vi "registerCommands.vi"(8 "error in (no error)":errorcluster, 11 "SAL_Listener in":refnum<class "SAL_Listener.lvclass">) -> (0 "error out":errorcluster, 3 "SAL_Listener out":refnum<class "SAL_Listener.lvclass">)   [LabVIEW 2016, in "SAL_Listener.lvclass"]
uses:
  SAL_Listener.lvclass
  SAL_Listener.lvclass/SAL_Listener.ctl
  SALLV_dome/SALLV_dome.lvlib
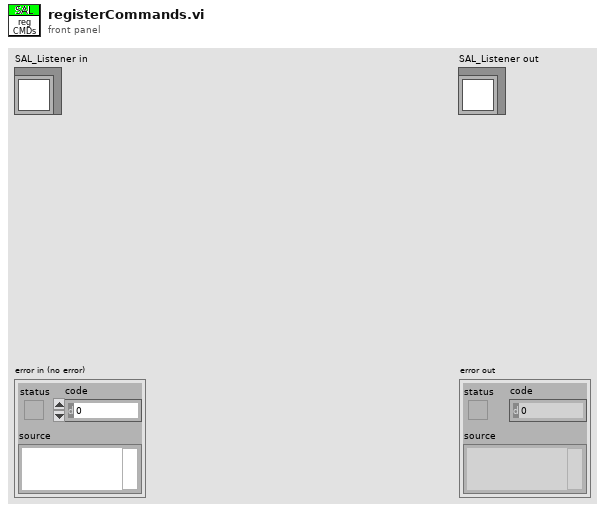
[diagram p1: front panel]
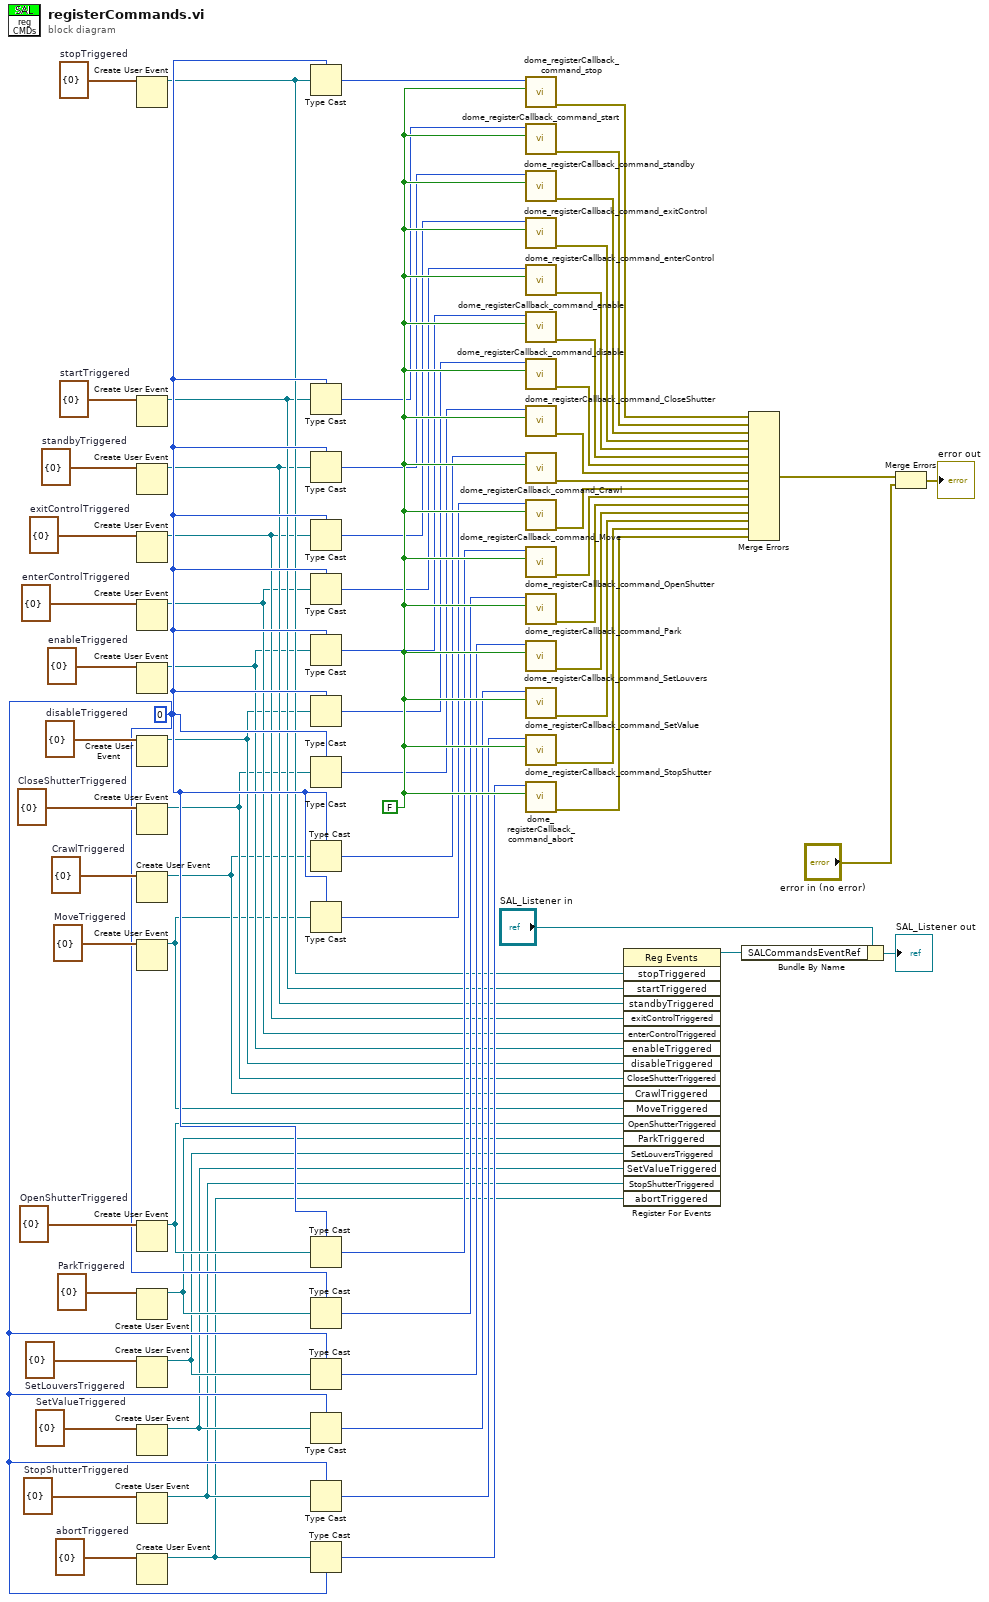
[diagram p0: block diagram]
diagram:
  w55 = 0 ("handle")
  w56 = FALSE
  w57 = cluster{"data":i32} {"data"=0}  # abortTriggered
  w59 = cluster{"data":i32} {"data"=0}  # SetValueTriggered
  w58 = cluster{"data":i32} {"data"=0}  # StopShutterTriggered
  w60 = cluster{"data":i32} {"data"=0}  # SetLouversTriggered
  w61 = cluster{"data":i32} {"data"=0}  # ParkTriggered
  w62 = cluster{"data":i32} {"data"=0}  # OpenShutterTriggered
  w63 = cluster{"data":i32} {"data"=0}  # MoveTriggered
  w64 = cluster{"data":i32} {"data"=0}  # CrawlTriggered
  w65 = cluster{"data":i32} {"data"=0}  # CloseShutterTriggered
  w66 = cluster{"data":i32} {"data"=0}  # disableTriggered
  w67 = cluster{"data":i32} {"data"=0}  # enableTriggered
  w68 = cluster{"data":i32} {"data"=0}  # enterControlTriggered
  w69 = cluster{"data":i32} {"data"=0}  # exitControlTriggered
  w70 = cluster{"data":i32} {"data"=0}  # standbyTriggered
  w71 = cluster{"data":i32} {"data"=0}  # startTriggered
  w72 = cluster{"data":i32} {"data"=0}  # stopTriggered
  n1 = Create User Event(user event datatype=w72) -> (user event=w19:refnum<user-event>)  [unwired: 1 in, 1 out]
  n2 = Create User Event(user event datatype=w71) -> (user event=w18:refnum<user-event>)  [unwired: 1 in, 1 out]
  n3 = Create User Event(user event datatype=w70) -> (user event=w17:refnum<user-event>)  [unwired: 1 in, 1 out]
  n4 = Create User Event(user event datatype=w69) -> (user event=w16:refnum<user-event>)  [unwired: 1 in, 1 out]
  n5 = Create User Event(user event datatype=w68) -> (user event=w15:refnum<user-event>)  [unwired: 1 in, 1 out]
  n6 = Create User Event(user event datatype=w67) -> (user event=w14:refnum<user-event>)  [unwired: 1 in, 1 out]
  n7 = Create User Event(user event datatype=w66) -> (user event=w13:refnum<user-event>)  [unwired: 1 in, 1 out]
  n8 = Create User Event(user event datatype=w65) -> (user event=w12:refnum<user-event>)  [unwired: 1 in, 1 out]
  n9 = Create User Event(user event datatype=w64) -> (user event=w11:refnum<user-event>)  [unwired: 1 in, 1 out]
  n10 = Create User Event(user event datatype=w63) -> (user event=w10:refnum<user-event>)  [unwired: 1 in, 1 out]
  n11 = Create User Event(user event datatype=w62) -> (user event=w9:refnum<user-event>)  [unwired: 1 in, 1 out]
  n12 = Create User Event(user event datatype=w61) -> (user event=w8:refnum<user-event>)  [unwired: 1 in, 1 out]
  n13 = Create User Event(user event datatype=w60) -> (user event=w7:refnum<user-event>)  [unwired: 1 in, 1 out]
  n14 = Create User Event(user event datatype=w59) -> (user event=w6:refnum<user-event>)  [unwired: 1 in, 1 out]
  n15 = Create User Event(user event datatype=w58) -> (user event=w5:refnum<user-event>)  [unwired: 1 in, 1 out]
  n16 = Create User Event(user event datatype=w57) -> (user event=w4:refnum<user-event>)  [unwired: 1 in, 1 out]
  n17 = Type Cast(type=w55, x=w19) -> (*(type *) &x=w54:i32)
  n18 = Type Cast(type=w55, x=w18) -> (*(type *) &x=w53:i32)
  n19 = Type Cast(type=w55, x=w17) -> (*(type *) &x=w52:i32)
  n20 = Type Cast(type=w55, x=w16) -> (*(type *) &x=w51:i32)
  n21 = Type Cast(type=w55, x=w15) -> (*(type *) &x=w50:i32)
  n22 = Type Cast(type=w55, x=w14) -> (*(type *) &x=w49:i32)
  n23 = Type Cast(type=w55, x=w13) -> (*(type *) &x=w48:i32)
  n24 = Type Cast(type=w55, x=w12) -> (*(type *) &x=w47:i32)
  n25 = Type Cast(type=w55, x=w11) -> (*(type *) &x=w46:i32)
  n26 = Type Cast(type=w55, x=w10) -> (*(type *) &x=w45:i32)
  n27 = Type Cast(type=w55, x=w9) -> (*(type *) &x=w44:i32)
  n28 = Type Cast(type=w55, x=w8) -> (*(type *) &x=w43:i32)
  n29 = Type Cast(type=w55, x=w7) -> (*(type *) &x=w42:i32)
  n30 = Type Cast(type=w55, x=w6) -> (*(type *) &x=w41:i32)
  n31 = Type Cast(type=w55, x=w5) -> (*(type *) &x=w40:i32)
  n32 = Type Cast(type=w55, x=w4) -> (*(type *) &x=w39:i32)
  n33 = call "dome_registerCallback_command_stop.vi"("skipOld"=w56, "handle"=w54) -> ("error out"=w20:errorcluster)  [unwired: 8 in, 1 out]
  n34 = call "dome_registerCallback_command_start.vi"("skipOld"=w56, "handle"=w53) -> ("error out"=w38:errorcluster)  [unwired: 8 in, 1 out]
  n35 = call "dome_registerCallback_command_standby.vi"("skipOld"=w56, "handle"=w52) -> ("error out"=w37:errorcluster)  [unwired: 8 in, 1 out]
  n36 = call "dome_registerCallback_command_exitControl.vi"("skipOld"=w56, "handle"=w51) -> ("error out"=w36:errorcluster)  [unwired: 8 in, 1 out]
  n37 = call "dome_registerCallback_command_enterControl.vi"("skipOld"=w56, "handle"=w50) -> ("error out"=w35:errorcluster)  [unwired: 8 in, 1 out]
  n38 = call "dome_registerCallback_command_enable.vi"("skipOld"=w56, "handle"=w49) -> ("error out"=w34:errorcluster)  [unwired: 8 in, 1 out]
  n39 = call "dome_registerCallback_command_disable.vi"("skipOld"=w56, "handle"=w48) -> ("error out"=w33:errorcluster)  [unwired: 8 in, 1 out]
  n40 = call "dome_registerCallback_command_CloseShutter.vi"("skipOld"=w56, "handle"=w47) -> ("error out"=w32:errorcluster)  [unwired: 8 in, 1 out]
  n41 = call "dome_registerCallback_command_Crawl.vi"("skipOld"=w56, "handle"=w46) -> ("error out"=w31:errorcluster)  [unwired: 8 in, 1 out]
  n42 = call "dome_registerCallback_command_Move.vi"("skipOld"=w56, "handle"=w45) -> ("error out"=w30:errorcluster)  [unwired: 8 in, 1 out]
  n43 = call "dome_registerCallback_command_OpenShutter.vi"("skipOld"=w56, "handle"=w44) -> ("error out"=w29:errorcluster)  [unwired: 8 in, 1 out]
  n44 = call "dome_registerCallback_command_Park.vi"("skipOld"=w56, "handle"=w43) -> ("error out"=w28:errorcluster)  [unwired: 8 in, 1 out]
  n45 = call "dome_registerCallback_command_SetLouvers.vi"("skipOld"=w56, "handle"=w42) -> ("error out"=w27:errorcluster)  [unwired: 8 in, 1 out]
  n46 = call "dome_registerCallback_command_SetValue.vi"("skipOld"=w56, "handle"=w41) -> ("error out"=w26:errorcluster)  [unwired: 8 in, 1 out]
  n47 = call "dome_registerCallback_command_StopShutter.vi"("skipOld"=w56, "handle"=w40) -> ("error out"=w25:errorcluster)  [unwired: 8 in, 1 out]
  n48 = call "dome_registerCallback_command_abort.vi"("skipOld"=w56, "handle"=w39) -> ("error out"=w24:errorcluster)  [unwired: 8 in, 1 out]
  n49 = register-events(w19, w18, w17, w16, w15, w14, w13, w12, w11, w10, w9, w8, w7, w6, w5, w4) -> (reference out=w1:refnum<event-registration>)  [unwired: 2 in, 1 out]
  n50 = Bundle By Name(cluster="SAL_Listener in", "SALCommandsEventRef"=w1) -> (→"SAL_Listener out":refnum<class "SAL_Listener.lvclass">)
  n51 = Merge Errors(w20, w38, w37, w36, w35, w34, w33, w32, w31, w30, w29, w28, w27, w26, w25, w24) -> (w21:errorcluster)
  n52 = Merge Errors(w21, "error in (no error)") -> (→"error out":errorcluster)
